vi "Configure relay channel.vi"(8 "error in (no error)":errorcluster, 10 "relay frequency":dbl[unit] format="%.6g", 11 "VISA resource name":refnum<visa-resource-name>="AFG3252") -> (0 "error out":errorcluster, 3 "VISA resource name out":refnum<visa-resource-name>)   [LabVIEW 2012]
doc: "Configures channel 2 of the AFG3252 (function generator) to output a series of three pulses, meant to control the relays. (To be used in conjunction with <B>Set FM sweep.vi<B>)"
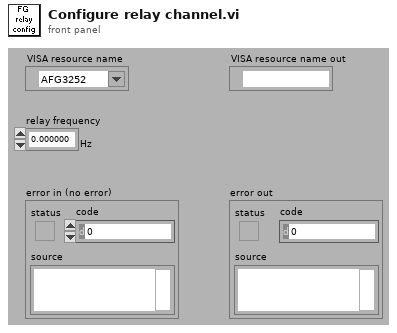
[diagram p1: front panel]
types:
  T1 = typedef "Semaphore RefNum" = refnum<k1>
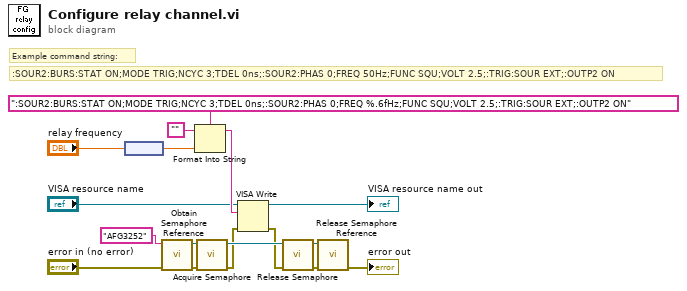
[diagram p0: block diagram]
diagram:
  # "Example command string:"
  # ":SOUR2:BURS:STAT ON;MODE TRIG;NCYC 3;TDEL 0ns;:SOUR2:PHAS 0;FREQ 50Hz;FUNC SQU;VOLT 2.5;:TRIG:SOUR EXT;:OUTP2 ON"
  n1 = node("relay frequency") -> (w5:dbl)
  n2 = call <vilib>:"Obtain Semaphore Reference.vi"("error in (no error)"="error in (no error)", "name (unnamed)"="AFG3252") -> ("error out"=w14:errorcluster, "semaphore"=w13:T1)  [unwired: 1 in, 3 out]
  n3 = Format Into String(format string=":SOUR2:BURS:STAT ON;MODE TRIG;NCYC 3;TDEL 0ns;:SOUR2:PHAS 0;FREQ %.6fHz;FUNC SQU;VOLT 2.5;:TRIG:SOUR EXT;:OUTP2 ON", initial string="", w5) -> (resulting string=w15:string)  [unwired: 1 in, 1 out]
  n4 = call <vilib>:"Acquire Semaphore.vi"("error in (no error)"=w14, "semaphore"=w13) -> ("error out"=w4:errorcluster, "semaphore out"=w8:T1)  [unwired: 1 in, 3 out]
  n5 = VISA Write(VISA resource name="VISA resource name", write buffer=w15, error in (no error)=w4) -> (VISA resource name out=→"VISA resource name out":refnum<visa-resource-name>, error out=w2:errorcluster)  [unwired: 1 out]
  n6 = call <vilib>:"Release Semaphore.vi"("error in (no error)"=w2, "semaphore"=w8) -> ("error out"=w10:errorcluster, "semaphore out"=w9:T1)  [unwired: 4 out]
  n7 = call <vilib>:"Release Semaphore Reference.vi"("error in (no error)"=w10, "semaphore"=w9) -> ("error out"=→"error out":errorcluster)  [unwired: 9 out]
